vi "LED Lights Subsystem.vi"(8 "error in":errorcluster) -> ()   [LabVIEW 2015]
uses:
  <vilib>/Rock Robotics/SystemInterfaces/i2clib/i2c_bus.ctl
  <vilib>/Rock Robotics/Network Tables/NT Read Boolean.vi
  LED Lights Global.vi
panel:
  in  "Send":bool
  in  "Light ID":u8=3
  in  "Blue":u8=153
  in  "Green":u8=12
  in  "Red":u8=64
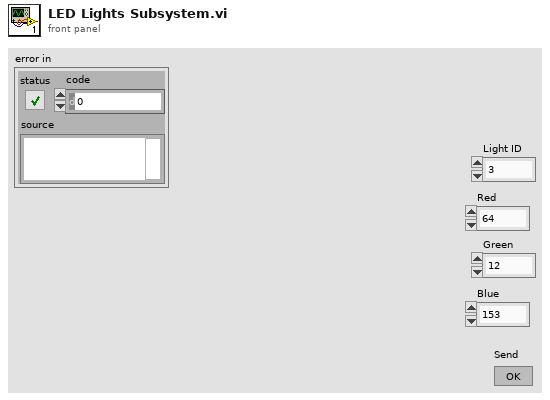
[diagram p1: front panel]
types:
  T1 = typedef "i2c_bus.ctl" = enum16{"I2C On-Board", "I2C MXP", "Invalid"}
  T2 = typedef "LED Lights Ref.ctl" = cluster{"I2CDevRef":T3}
  T3 = typedef "WPI_I2CDevRef.ctl" = cluster{"DevStatus":errorcluster, "Device Address":u8, "Handle":i32, "I2C Bus":T1}
  T4 = typedef "NavX Light Global Type Def.ctl" = cluster{"NavX Error":errorcluster, "Initialized":bool}
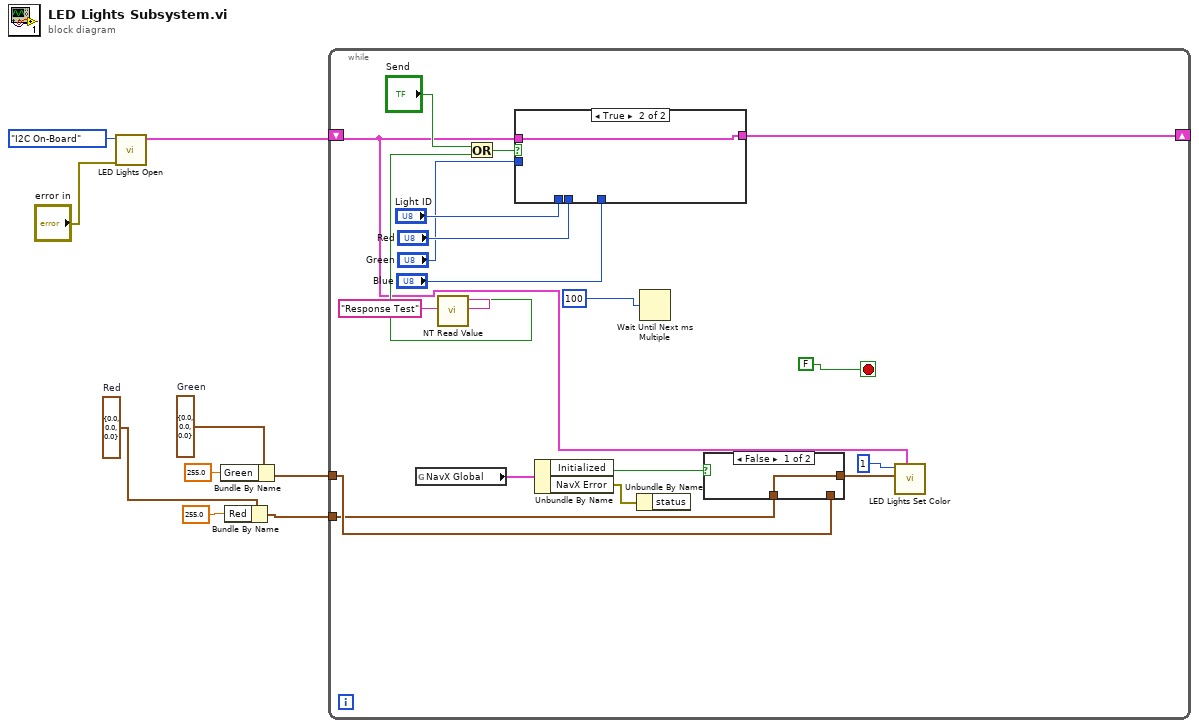
[diagram p0: block diagram]
diagram:
  w3 = cluster{"Red":dbl, "Green":dbl, "Blue":dbl} {"Red"=0.0, "Green"=0.0, "Blue"=0.0}  # Red
  w6 = cluster{"Red":dbl, "Green":dbl, "Blue":dbl} {"Red"=0.0, "Green"=0.0, "Blue"=0.0}  # Green
  n1 = call "LED Lights Open.vi"("error in"="error in", "I2C Bus"=i2c_bus."I2C On-Board") -> ("output cluster"=w7:T2)  [unwired: 8 in, 1 out]
  n2 = Bundle By Name(cluster=w6, "Green"=255.0) -> (w4:cluster{"Red":dbl, "Green":dbl, "Blue":dbl})
  n3 = Bundle By Name(cluster=w3, "Red"=255.0 ("Green")) -> (w1:cluster{"Red":dbl, "Green":dbl, "Blue":dbl})
  n4 = while {
    shift-right: [w22] -> _
    shift-left: w7 -> [w16]
    tunnel: w4 -> [w12]
    tunnel: w1 -> [w11]
    stop <- FALSE stop-if-true
    n5 = global read "LED Lights Global.vi" "NavX Global"() -> (w10:T4)
    n6 = call-poly <vilib>:"NT Read Value.vi"("Name"="Response Test") -> ("Boolean"=w18:bool)  [unwired: 9 in, 1 out]
    n7 = Or(x="Send", y=w18) -> (x .or. y?=w21:bool)
    n8 = case shown="True" w21 {
      tunnel: w16 -> [w31 w32]
      tunnel: "Light ID" -> [_ _]
      tunnel: "Red" -> [_ _]
      tunnel: "Green" -> [_ _]
      tunnel: "Blue" -> [_ _]
      tunnel: [w31 w32] -> w22
      frame False {
      }
      frame True {
      }
    }
    n9 = Unbundle By Name(w10) -> ("Initialized"=w14:bool, "NavX Error"=w17:errorcluster)
    n10 = Unbundle By Name(w17) -> ()  [unwired: 1 out]
    n11 = Wait Until Next ms Multiple(millisecond multiple=100) -> ()  [unwired: 1 out]
    n12 = case shown="False" w14 {
      tunnel: [w29 w30] -> w13
      tunnel: w12 -> [_ w30]
      tunnel: w11 -> [w29 _]
      frame False {
      }
      frame True {
      }
    }
    n13 = call "LED Lights Set Color.vi"("LED Lights Ref In"=w16, "Color"=w13, "Light ID"=u8 1 ("Light ID 2")) -> ()  [unwired: 7 in, 2 out]
  }
